vi "writeEndOfFrame.vi"(8 "error in (no error)":errorcluster, 11 "ModbusBuffer in":refnum<class "ModbusBufferBuilder.lvclass">) -> (0 "error out":errorcluster, 3 "ModbusBuffer out":refnum<class "ModbusBufferBuilder.lvclass">)   [LabVIEW 2016, in "ModbusBufferBuilder.lvclass"]
uses:
  ModbusBufferBuilder.lvclass
  ModbusBufferBuilder.lvclass/ModbusBufferBuilder.ctl
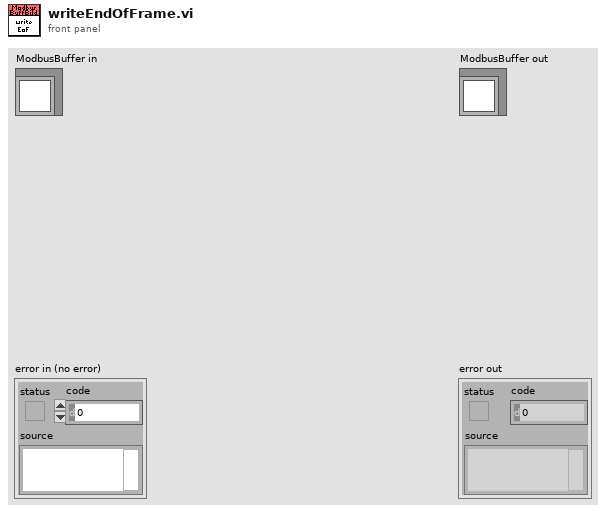
[diagram p1: front panel]
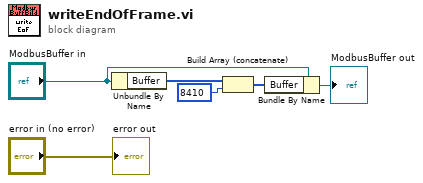
[diagram p0: block diagram]
diagram:
  n1 = Unbundle By Name("ModbusBuffer in") -> ("Buffer"=w3:u16[])
  n2 = Build Array (concatenate)(w3, u16 8410 ("x")) -> (w2:u16[])
  n3 = Bundle By Name(cluster="ModbusBuffer in", "Buffer"=w2) -> (→"ModbusBuffer out":refnum<class "ModbusBufferBuilder.lvclass">)
  "error out" <- "error in (no error)"
